vi "Pcre2GetErrorMessage8.vi"(8 "error in":errorcluster, 11 "ErrorCode":i32) -> (0 "error out":errorcluster, 2 "ErrorMessage":string, 3 "return":i32)   [LabVIEW 2021, in "libpcre2-8.lvlib"]
uses:
  libpcre2-8.lvlib
  libpcre2-8-x32.dll
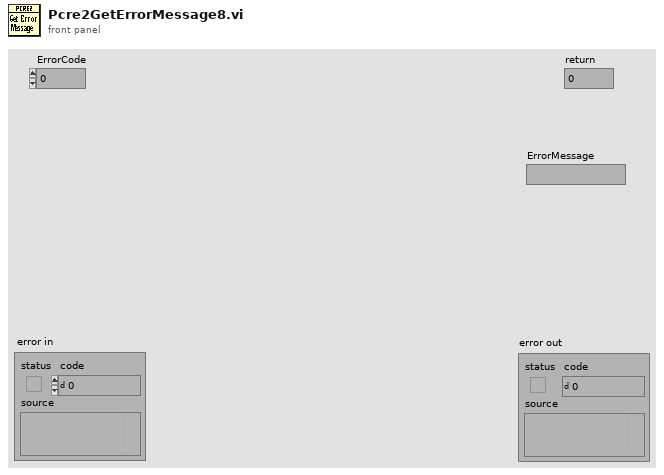
[diagram p1: front panel]
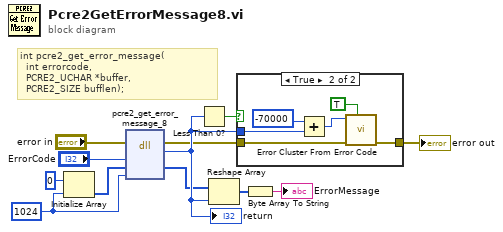
[diagram p0: block diagram]
diagram:
  w1 = u64 1024 ("bufflen")
  # "int pcre2_get_error_message(\n  int errorcode, \n  PCRE2_UCHAR *buffer, \n  PCRE2_SIZE bufflen);"
  n1 = Initialize Array(u8 0 ("U8"), w1) -> (w7:u8[])
  n2 = dll-call lib="libpcre2-8-x*.dll" fn="pcre2_get_error_message_8"(error in="error in", "errorcode"="ErrorCode", "buffer"=w7, "bufflen"=w1) -> (error out=w3:errorcluster, "return"=w9:i32, "buffer"=w6:u8[])  [unwired: 4 in, 1 out]
  "return" <- w9
  n3 = Less Than 0?(x=w9) -> (x < 0?=w4:bool)
  n4 = Reshape Array(w6, w9) -> (w5:u8[])
  n5 = case shown="True" w4 {
    tunnel: w3 -> [w13 w16]
    tunnel: [w13 w15] -> w10
    tunnel: w9 -> [_ w18]
    frame False {
    }
    frame True {
      n6 = Add(x=-70000 ("errorcode"), y=w18) -> (x+y=w17:i32)
      n7 = call <vilib>:"Error Cluster From Error Code.vi"("show call chain? (False)"=TRUE, "error in (no error)"=w16, "error code (0)"=w17) -> ("error out"=w15:errorcluster)  [unwired: 6 in]
    }
  }
  "error out" <- w10
  n8 = Byte Array To String(unsigned byte array=w5) -> (string=→"ErrorMessage":string)
